vi "Data Memory Operation.vi"(8 "error in (no error)":errorcluster, 10 "Memory Operation (0: Fill)":u16(ring) items=["Fill", "Read", "Clear"], 11 "VISA resource name":refnum<visa-resource-name>) -> (0 "error out":errorcluster, 3 "VISA resource name out":refnum<visa-resource-name>)   [LabVIEW 2017, in "Agilent E4980.lvlib"]
doc: "The data buffer memory operations include:\n \n(1) Enables the data buffer memory to store measurement data.\n(2) Places the data in the buffer memory into the output buffer.\n(3) Clears and disables the data buffer memory."
uses:
  Agilent E4980.lvlib
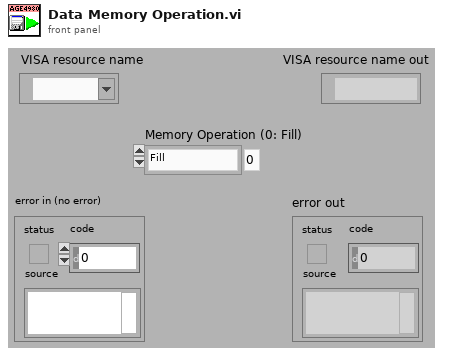
[diagram p1: front panel]
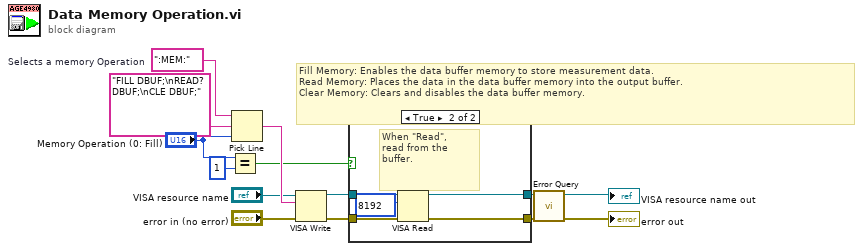
[diagram p0: block diagram]
diagram:
  w2 = "FILL DBUF;\nREAD? DBUF;\nCLE DBUF;"  # Selects a memory Operation
  # "Fill Memory: Enables the data buffer memory to store measurement data.\nRead Memory: Places the data in the data buffer memory into the output buffer.\nClear Memory: Clears and disables the data buffer memory."
  n1 = Equal?(x="Memory Operation (0: Fill)", y=u16 1) -> (x = y?=w7:bool)
  n2 = Pick Line(string ("")=":MEM:", multi-line string=w2, line index="Memory Operation (0: Fill)") -> (output string=w12:string)
  n3 = VISA Write(VISA resource name="VISA resource name", write buffer=w12, error in (no error)="error in (no error)") -> (VISA resource name out=w6:refnum<visa-resource-name>, error out=w5:errorcluster)  [unwired: 1 out]
  n4 = case shown="True" w7 {
    tunnel: w6 -> [w16 w21]
    tunnel: w5 -> [w15 w20]
    tunnel: [w16 w19] -> w4
    tunnel: [w15 w18] -> w3
    frame False {
      # "Execute the command,\nread nothing."
    }
    frame True {
      # "When \"Read\",\nread from the\nbuffer."
      n5 = VISA Read(VISA resource name=w21, byte count=u32 8192, error in (no error)=w20) -> (VISA resource name out=w19:refnum<visa-resource-name>, error out=w18:errorcluster)  [unwired: 2 out]
    }
  }
  n6 = call "Error Query.vi"("error in (no error)"=w3, "VISA resource name"=w4) -> ("error out"=→"error out":errorcluster, "VISA resource name out"=→"VISA resource name out":refnum<visa-resource-name>)  [unwired: 6 in, 2 out]
